vi "Get VI From Class.vi"(0 "Class Library":refnum<vi>, 5 "Class Item Name":string, 11 "error in":errorcluster) -> (4 "Class Library":refnum<vi>, 8 "Class Item Refnum":refnum<vi>, 15 "error out":errorcluster)   [LabVIEW 2012, in "REx_Springboard.lvlib"]
uses:
  REx_Springboard.lvlib
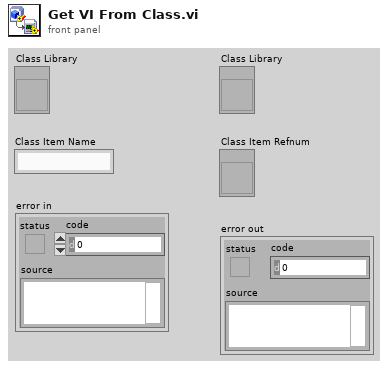
[diagram p1: front panel]
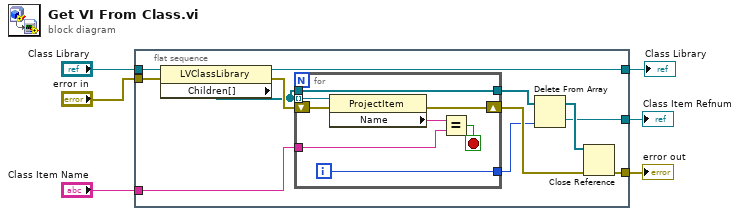
[diagram p0: block diagram]
diagram:
  n1 = flat-sequence {
    tunnel: "error in" -> [w16]
    tunnel: "Class Library" -> [w15]
    tunnel: [w12] -> w2
    tunnel: [w11] -> w3
    tunnel: [w10] -> w4
    tunnel: "Class Item Name" -> [w9]
    frame #0 {
      n2 = property class="LVClassLibrary"(reference=w15, error in=w16) -> (reference out=w10:refnum<vi>, error out=w17:errorcluster, "Children[]"=w8:refnum<vi>[])
      n3 = for {
        tunnel: w8 -> [w26] mode=indexing
        tunnel: w9 -> [w24]
        tunnel: [w23] -> w14
        shift-right: [w20] -> w18
        shift-left: w17 -> [w21]
        tunnel: [w19] -> w7
        tunnel: w8 -> [w19]
        i -> [w23]
        stop <- w22 stop-if-true
        n4 = property class="ProjectItem"(reference=w26, error in=w21) -> (error out=w20:errorcluster, "Name"=w25:string)  [unwired: 1 out]
        n5 = Equal?(x=w25, y=w24) -> (x = y?=w22:bool)
      }
      n6 = Delete From Array(array=w7, index=w14) -> (deleted portion=w12:refnum<vi>, array with subset deleted=w13:refnum<vi>[])  [unwired: 1 in]
      n7 = Close Reference(reference=w13, error in (no error)=w18) -> (error out=w11:errorcluster)
    }
  }
  "Class Library" <- w4
  "error out" <- w3
  "Class Item Refnum" <- w2
